vi "VCS Get Velocity Profile.vi"(8 "error in (no error)":errorcluster, 11 "axis in":cluster{"keyHandle":u32, "nodeId":u16}={"keyHandle"=0, "nodeId"=1}) -> (0 "error out":errorcluster, 2 "velocity profile":T1, 3 "axis out":cluster{"keyHandle":u32, "nodeId":u16}={"keyHandle"=0, "nodeId"=1})   [LabVIEW 2010]
doc: "<B>VCS Get Velocity Profile</B> returns the velocity profile parameters."
uses:
  Resources/EposCmd.dll
  Resources/EposCmd64.dll
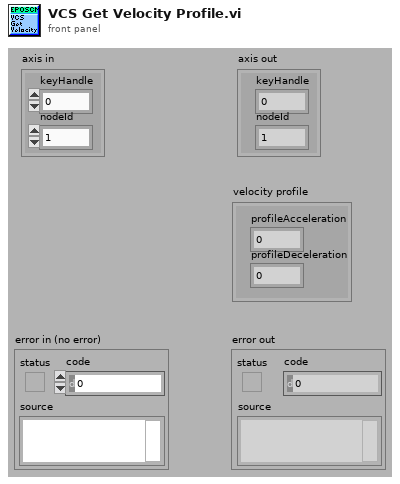
[diagram p1: front panel]
types:
  T1 = cluster{"profileAcceleration":u32, "profileDeceleration":u32}
  T2 = cluster{"pProfileAcceleration":u32, "pProfileDeceleration":u32}
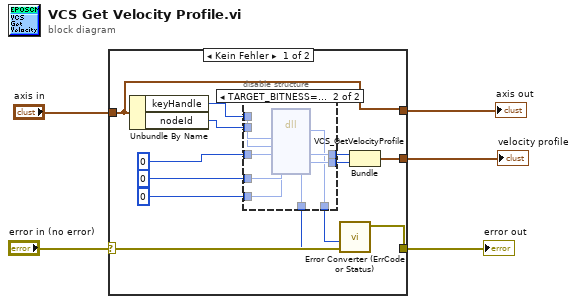
[diagram p0: block diagram]
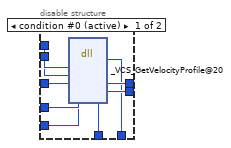
[diagram p2: hidden frame]
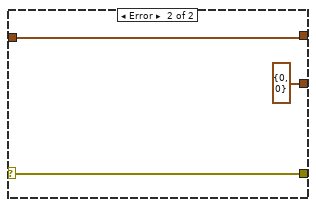
[diagram p3: hidden frame]
diagram:
  n1 = case shown="Kein Fehler" "error in (no error)" {
    selector: "error in (no error)" -> [w18 w39]
    tunnel: [w17 w39] -> w4
    tunnel: "axis in" -> [w7 w38]
    tunnel: [w8 T2 {"pProfileAcceleration"=0, "pProfileDeceleration"=0}] -> w1
    tunnel: [w7 w38] -> w2
    frame No Error {
      n2 = Unbundle By Name(w7) -> ("keyHandle"=w15:u32, "nodeId"=w14:u16)
      n3 = disable-structure shown="TARGET_BITNESS==64" {
        disable-tunnel: [w27 w36] -> w16
        disable-tunnel: w15 -> [w26 w35]
        disable-tunnel: w14 -> [w25 w34]
        disable-tunnel: u32 0 ("pProfileAcceleration") -> [w24 w33]
        disable-tunnel: u32 0 ("pProfileDeceleration") -> [w23 w32]
        disable-tunnel: u32 0 ("pErrorCode") -> [w22 w31]
        disable-tunnel: [w21 w30] -> w10
        disable-tunnel: [w20 w29] -> w9
        disable-tunnel: [w19 w28] -> w6
        frame condition #0 (active) {
          n4 = dll-call lib="C:/Sources/LabView/maxon EPOS/Resources/EposCmd.*" fn="_VCS_GetVelocityProfile@20"("KeyHandle"=w26, "NodeId"=w25, "pProfileAcceleration"=w24, "pProfileDeceleration"=w23, "pErrorCode"=w22) -> (w19:i32, "pProfileAcceleration"=w21:u32, "pProfileDeceleration"=w20:u32, "pErrorCode"=w27:u32)  [unwired: 5 in, 2 out]
        }
        frame condition #1 {
          n5 = dll-call lib="C:/LabVIEW/maxon EPOS/Resources/EposCmd64.dll" fn="VCS_GetVelocityProfile" ("EposCmd.dll:_VCS_GetVelocityProfile@20")("KeyHandle"=w35, "NodeId"=w34, "pProfileAcceleration"=w33, "pProfileDeceleration"=w32, "pErrorCode"=w31) -> ("Rückgabetyp"=w28:i32, "pProfileAcceleration"=w30:u32, "pProfileDeceleration"=w29:u32, "pErrorCode"=w36:u32)  [unwired: 5 in, 2 out]
        }
      }
      n6 = call "Error Converter (ErrCode or Status).vi"("error code"=w16, "return type"=w6, "error in (no error)"=w18) -> ("error out"=w17:errorcluster)  [unwired: 7 in]
      n7 = Bundle("pProfileAcceleration"=w10, "pProfileDeceleration"=w9) -> (w8:T2)  [unwired: 1 in]
    }
    frame Error {
    }
  }
  "error out" <- w4
  "axis out" <- w2
  "velocity profile" <- w1
